vi "Grid To Bool Array.vi"(8 "error in (no error)":errorcluster, 10 "Bool Array In":bool[](array[boolean]), 11 "ElectrodeGrid in":refnum<class "ElectrodeGrid.lvclass">) -> (0 "error out":errorcluster, 2 "Bool Array Out":bool[](array[boolean]), 3 "ElectrodeGrid out":refnum<class "ElectrodeGrid.lvclass">)   [LabVIEW 2017, in "ElectrodeGrid.lvclass"]
uses:
  ElectrodeGrid.lvclass
  ElectrodeGrid.lvclass/ElectrodeGrid.ctl
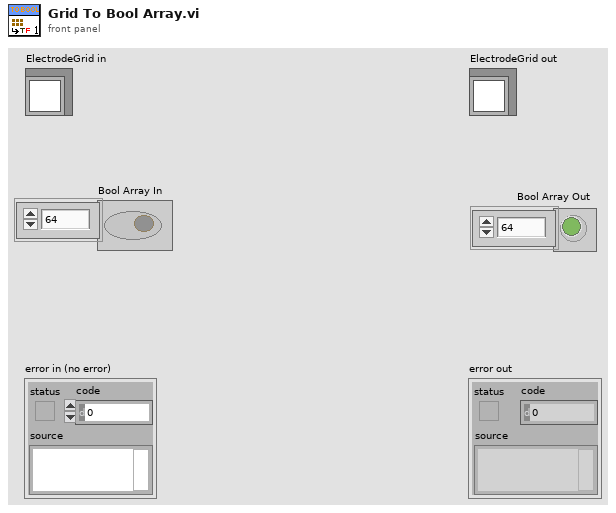
[diagram p1: front panel]
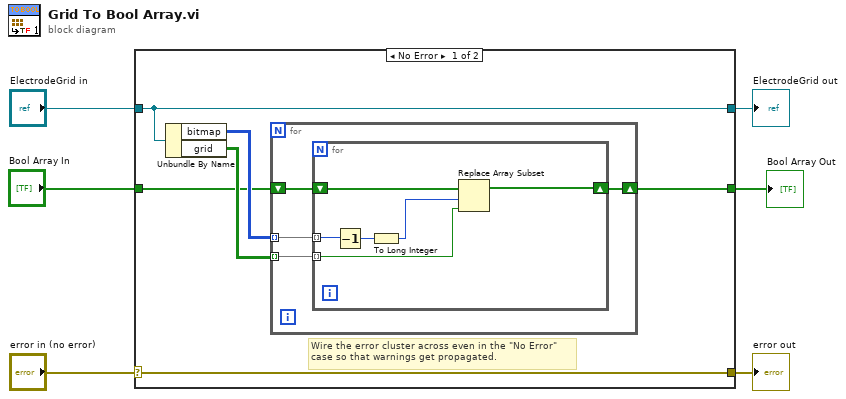
[diagram p0: block diagram]
diagram:
  n1 = case shown="No Error" "error in (no error)" {
    selector: "error in (no error)" -> [w12 w25]
    tunnel: [w12 w25] -> w5
    tunnel: [w11 w24] -> w3
    tunnel: "ElectrodeGrid in" -> [w11 w24]
    tunnel: "Bool Array In" -> [w8 w23]
    tunnel: [w7 w23] -> w1
    frame No Error {
      # "Wire the error cluster across even in the \"No Error\"\ncase so that warnings get propagated."
      n2 = Unbundle By Name(w11) -> ("bitmap"=w9:u8[][], "grid"=w10:bool[][])
      n3 = for {
        tunnel: w10 -> [w15] mode=indexing
        tunnel: w9 -> [w16] mode=indexing
        shift-right: [w13] -> w7
        shift-left: w8 -> [w14]
        n4 = for {
          tunnel: w16 -> [w22] mode=indexing
          tunnel: w15 -> [w19] mode=indexing
          shift-right: [w17] -> w13
          shift-left: w14 -> [w18]
          n5 = Decrement(x=w22) -> (x-1=w21:u8)
          n6 = To Long Integer(number=w21) -> (32bit integer=w20:i32)
          n7 = Replace Array Subset(array=w18, new element=w19, index=w20) -> (w17:bool[])
        }
      }
    }
    frame Error {
    }
  }
  "error out" <- w5
  "ElectrodeGrid out" <- w3
  "Bool Array Out" <- w1
